vi "Query Option Version Info.vi"(8 "error in (no error)":errorcluster, 10 "Application (\"\")":string, 11 "VISA resource name":refnum<visa-resource-name>) -> (0 "error out":errorcluster, 2 "System Installed Options List":string, 3 "VISA resource name out":refnum<visa-resource-name>)   [LabVIEW 2015, in "Rohde&Schwarz CMXP Base.lvlib"]
doc: "Returns version information for installed software packages. You can either query a list of all installed packages and their versions or you can query the version of a single package specified via <Application>: <Application> specified: A string is returned, indicating the version of the <Application>. If the specified <Application> is unknown / not installed, \"0\" is returned.<Application> omitted: A string is returned, containing a list of all installed software packages and their version in the format \"<PackageName1>,<Version1>;<PackageName2>,<Version2>;...\"\n\nAttribute:\n-\n\nRemote-control command:\nSYSTem:BASE:OPTion:VERSion?"
uses:
  <instrlib>/Rohde&Schwarz CMXP Base/Rohde&Schwarz CMXP Base.lvlib
  <instrlib>/Rohde&Schwarz CMXP Base/Private/rsidr_core.llb/rsidr_core.lvlib
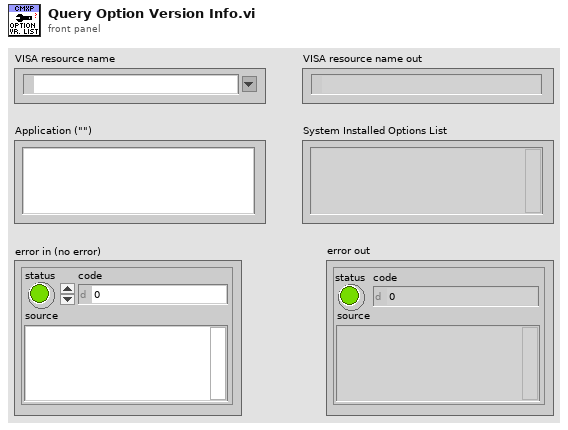
[diagram p1: front panel]
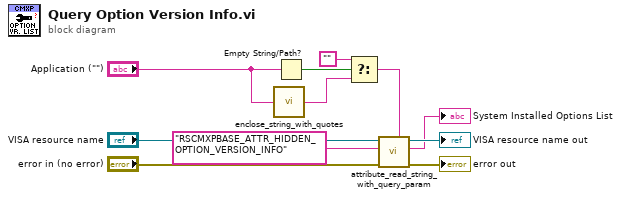
[diagram p0: block diagram]
diagram:
  n1 = call <instrlib>:"enclose_string_with_quotes.vi"("String to enclose"="Application (\"\")") -> ("String out"=w1:string)  [unwired: 4 in]
  n2 = Empty String/Path?(string/path="Application (\"\")") -> (empty?=w6:bool)
  n3 = Select(t="" ("Empty String Constant"), s=w6, f=w1) -> (s? t:f=w4:string)
  n4 = call <instrlib>:"attribute_read_string_with_query_param.vi"("Query Parameter (None)"=w4, "error in"="error in (no error)", "Attribute ID"="RSCMXPBASE_ATTR_HIDDEN_OPTION_VERSION_INFO", "VISA resource name"="VISA resource name") -> ("error out"=→"error out":errorcluster, "String out"=→"System Installed Options List":string, "VISA resource name out"=→"VISA resource name out":refnum<visa-resource-name>)  [unwired: 5 in]
